vi "报警交互入队列.vi"(8 "错误输入（无错误）":errorcluster, 9 "告警内容":string, 10 "告警码":string, 11 "报警模块":string) -> (0 "错误输出":errorcluster)   [LabVIEW 2016, in "斯坦道氨氮.lvlib"]
panel:
  out "输出簇":T1
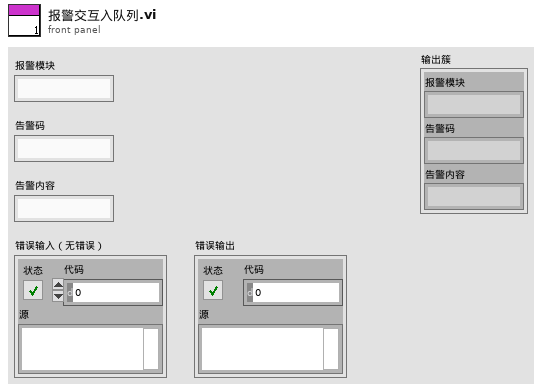
[diagram p1: front panel]
types:
  T1 = cluster{"报警模块":string, "告警码":string, "告警内容":string}
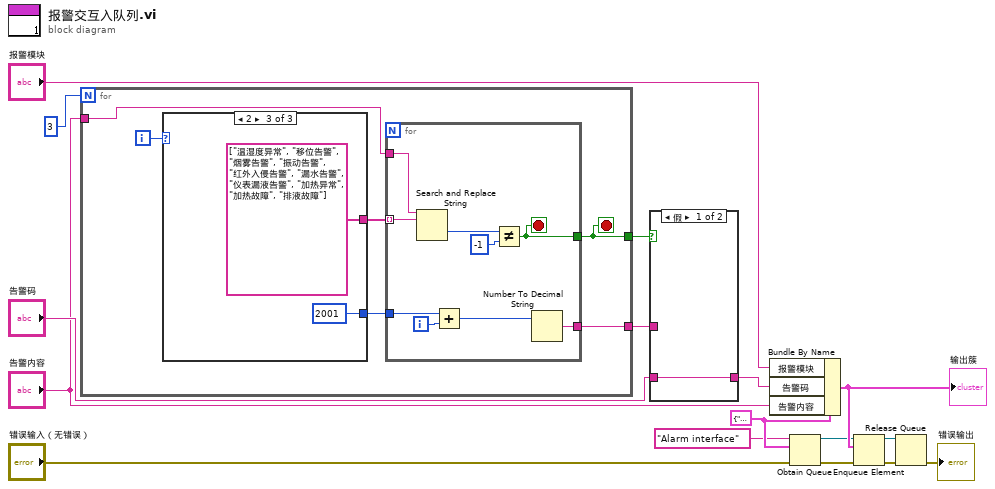
[diagram p0: block diagram]
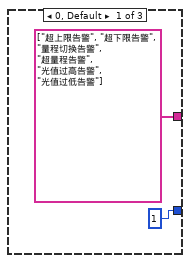
[diagram p3: hidden frame]
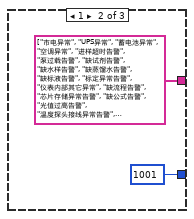
[diagram p4: hidden frame]
diagram:
  w14 = T1 {"报警模块"="", "告警码"="", "告警内容"=""}
  n1 = for {
    N: 3 -> [_]
    tunnel: "告警内容" -> [w22]
    tunnel: [w21] -> w4
    tunnel: [w17] -> w5
    i -> [w20]
    stop <- w17 stop-if-true
    n2 = case shown="2" w20 {
      tunnel: [1 ("x") 1001 ("x") 2001 ("x")] -> w19
      tunnel: [string[] ["超上限告警", "超下限告警", "量程切换告警", "超量程告警", "光值过高告警", "光值过低告警"] ("转置的数组") string[] ["市电异常", "UPS异常", "蓄电池异常", "空调异常", "进样超时告警", "泵过载告警", "缺试剂告警", "缺水样告警", "缺蒸馏水告警", "缺标液告警", "标定异常告警", "仪表内部其它异常", "缺流程告警", "芯片存储异常告警", "缺公式告警", "光值过高告警", "温度探头接线异常告警", "温度探头未嵌入凹槽或消解模块气密性差", "温度探头功率过大告警", "注射泵供电告警", "注射泵丝杆过载告警", "注射泵阀头切换过载告警", "注射泵配置异常告警", "注射泵通信异常告警", "光谱仪通信异常告警", "电机故障", "光路系统故障", "滴定异常告警", "缺高锰酸钾告警", "缺草酸钠告警", "缺硫酸告警", "ORP值异常告警", "A值异常告警", "B值异常告警", "环境温度传感器告警", "注射泵保温温度异常告警", "注射泵保温加热超时告警", "注射泵初始化异常告警", "注射泵运行超时告警", "加热温度超限告警", "加热或降温超时告警", "注射泵故障", "ORP故障", "偏心轮故障", "缺试剂检测故障", "缺零点样告警", "缺跨度样告警", "缺空白样告警", "缺平行样告警", "缺加标样告警", "缺试剂A", "缺试剂B", "水样余量过低", "标液余量过低", "零点样余量过低", "跨度样余量过低", "空白样余量过低", "平行样余量过低", "加标样余量过低", "试剂A余量过低", "试剂B余量过低", "请注意查看溶液或试剂余量并及时维护", "旋转阀通信异常告警", "旋转阀故障", "光路系统故障", "液位异常告警", "柱塞泵故障告警", "流程中断告警"] ("转置的数组") string[] ["温湿度异常", "移位告警", "烟雾告警", "振动告警", "红外入侵告警", "漏水告警", "仪表漏液告警", "加热异常", "加热故障", "排液故障"] ("转置的数组")] -> w18
      frame 0, Default {
      }
      frame 1 {
      }
      frame 2 {
      }
    }
    n3 = for {
      tunnel: w22 -> [w37]
      tunnel: w18 -> [w36] mode=indexing
      tunnel: [w32] -> w21
      tunnel: w19 -> [w30]
      tunnel: [w29] -> w17
      i -> [w31]
      stop <- w29 stop-if-true
      n4 = Search and Replace String(input string=w37, search string=w36) -> (offset past replacement=w35:i32)  [unwired: 6 in, 3 out]
      n5 = Add(x=w30, y=w31) -> (x+y=w33:i32)
      n6 = Not Equal?(x=w35, y=-1) -> (x != y?=w29:bool)
      n7 = Number To Decimal String(number=w33) -> (decimal integer string=w32:string)  [unwired: 1 in]
    }
  }
  n8 = case shown="假" w5 {
    tunnel: w4 -> [_ w39]
    tunnel: [w38 w39] -> w3
    tunnel: "告警码" -> [w38 _]
    frame False {
    }
    frame True {
    }
  }
  n9 = Bundle By Name(cluster=w14, "报警模块"="报警模块", "告警码"=w3, "告警内容"="告警内容") -> (w15:T1)
  "输出簇" <- w15
  n10 = Obtain Queue(name (unnamed)="Alarm interface" ("名称（未命名）"), element data type=w14, error in (no error)="错误输入（无错误）") -> (queue out=w10:refnum<queue>, error out=w11:errorcluster)  [unwired: 2 in, 1 out]
  n11 = Enqueue Element(queue=w10, element=w15, error in (no error)=w11) -> (queue out=w12:refnum<queue>, error out=w13:errorcluster)  [unwired: 1 in, 1 out]
  n12 = Release Queue(queue=w12, error in (no error)=w13) -> (error out=→"错误输出":errorcluster)  [unwired: 1 in, 2 out]
